vi "finish_transaction.vi"(0 "DB Session ID":i32, 11 "error in (no error)":errorcluster) -> (4 "DB Session ID out":i32, 15 "error out":errorcluster)   [LabVIEW 2017, in "Database.lvlib"]
uses:
  Database.lvlib
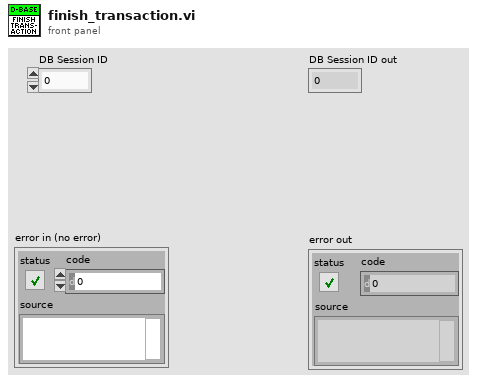
[diagram p1: front panel]
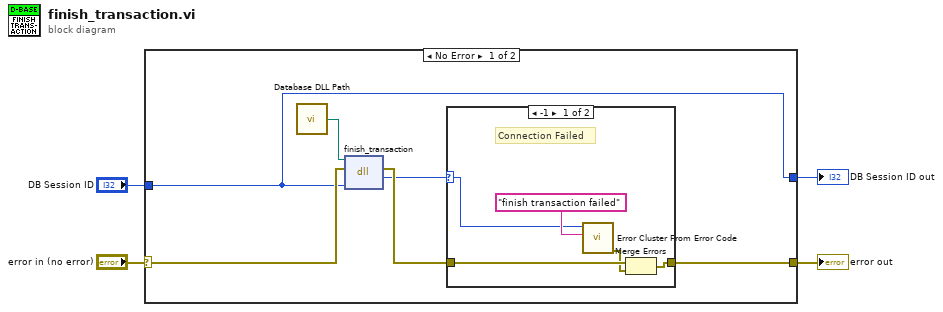
[diagram p0: block diagram]
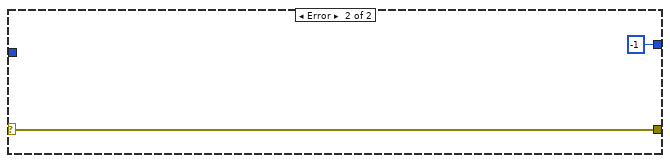
[diagram p3: hidden frame]
diagram:
  n1 = case shown="No Error" "error in (no error)" {
    selector: "error in (no error)" -> [w10 w18]
    tunnel: [w8 w18] -> w3
    tunnel: [w5 -1 ("return type")] -> w2
    tunnel: "DB Session ID" -> [w5 _]
    frame No Error {
      n2 = call "Database DLL Path.vi"() -> ("DLL Path"=w7:path)  [unwired: 5 in]
      n3 = dll-call lib="?" fn="finish_transaction"(path in=w7, error in=w10, "conn_id"=w5) -> (error out=w9:errorcluster, "return type"=w6:i32)  [unwired: 2 in, 1 out]
      n4 = case shown="-1" w6 {
        selector: w6 -> [w11 _]
        tunnel: w9 -> [w15 w16]
        tunnel: [w14 w16] -> w8
        frame -1 {
          # "Connection Failed"
          n5 = call <vilib>:"Error Cluster From Error Code.vi"("error message (\"\")"="finish transaction failed" ("error message (\"\")"), "error code (0)"=w11) -> ("error out"=w13:errorcluster)  [unwired: 7 in]
          n6 = Merge Errors(w15, w13) -> (w14:errorcluster)
        }
        frame Default {
        }
      }
    }
    frame Error {
    }
  }
  "error out" <- w3
  "DB Session ID out" <- w2
